vi "Load Voltage Measurement T11.vi"(0 "Device Name":refnum<k15>="Dev1", 7 "Range":dbl=10.0 format="%.2f", 9 "Resolution in Digits":T1=5.5 items=["3 1/2"=3.5, "4 1/2"=4.5, "5 1/2"=5.5, "6 1/2"=6.5, "7 1/2"=7.5], 11 "error in":errorcluster caption="error in (no error)") -> (4 "Measurement":T2 format="%.6p", 6 "Signal Out of Range":bool, 15 "error out":errorcluster)   [LabVIEW 2021, in "DMM t11.lvlib"]
doc: "This example acquires a single measurement from a National Instruments DMM. Select the measurement function and range. Specify the resolution in digits of precision. The measured value will be displayed in the Measurement indicator. The Boolean indicator will indicate if the measured value is out of range."
uses:
  DMM/DMM t11.lvlib
  controls/Measurement Result.ctl
  <instrlib>/niDMM/nidmm.llb/niDMM Resolution in Digits.ctl
  <instrlib>/niDMM/nidmm.llb/niDMM Function.ctl
  <instrlib>/niDMM/nidmm.llb/niDMM Configure Measurement Digits.vi
  Reusables/Resuables T11.lvlib
panel:
  # "For instructions select File >> VI Properties >> Documentation"
  # "Configuration"
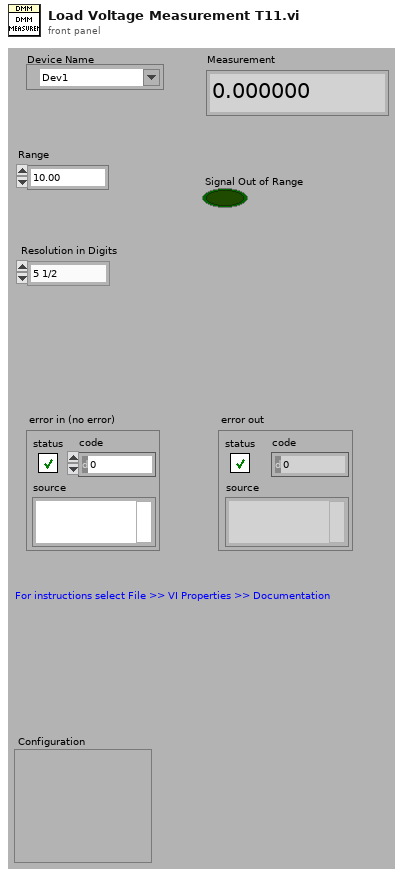
[diagram p1: front panel]
types:
  T1 = typedef "niDMM Resolution in Digits.ctl" = dbl
  T2 = typedef "Resuables T11.lvlib/Measurement Result.ctl" = dbl
  T3 = typedef "niDMM Function.ctl" = enum16{"DC Volts", "AC Volts", "DC Current", "AC Current", "2-wire Resistance", "4-wire Resistance", "Diode", "Frequency", "Period", "AC Volts DC Coupled", "Capacitance", "Inductance", "Temperature"}
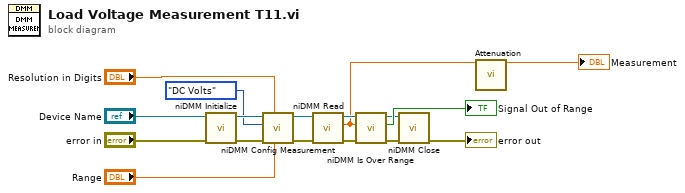
[diagram p0: block diagram]
diagram:
  n1 = call <instrlib>:"niDMM Initialize.vi"("error in (no error)"="error in", "Instrument Descriptor"="Device Name") -> ("error out"=w7:errorcluster, "instrument handle out"=w6:refnum<k15>)  [unwired: 8 in]
  n2 = call-poly <instrlib>:"niDMM Config Measurement.vi"("Range"="Range", "Resolution in Digits"="Resolution in Digits", "error in (no error)"=w7, "Function"=niDMM_Function."DC Volts", "instrument handle"=w6) -> ("error out"=w11:errorcluster, "instrument handle out"=w10:refnum<k15>)  [unwired: 5 in]
  n3 = call <instrlib>:"niDMM Read.vi"("error in (no error)"=w11, "instrument handle"=w10) -> ("error out"=w8:errorcluster, "Measurement"=w2:dbl, "instrument handle out"=w9:refnum<k15>)  [unwired: 7 in]
  n4 = call <instrlib>:"niDMM Is Over Range.vi"("error in (no error)"=w8, "Measurement"=w2, "instrument handle"=w9) -> ("error out"=w4:errorcluster, "Over Range?"=→"Signal Out of Range":bool, "instrument handle out"=w5:refnum<k15>)  [unwired: 6 in]
  n5 = call <instrlib>:"niDMM Close.vi"("error in (no error)"=w4, "instrument handle"=w5) -> ("error out"=→"error out":errorcluster)  [unwired: 9 in]
  n6 = call "Attenuation.vi"("Measurement"=w2) -> ("Measurement Out"=→"Measurement":T2)  [unwired: 14 in]
